vi "SinglePoint-RemoveResultChannel.vi"(8 "Error in":errorcluster, 11 "Custom Device ref":T1 format="%.0x") -> (0 "Error out":errorcluster, 3 "Custom Device ref out":T1 format="%.0x")   [LabVIEW 2017, in "Waveform-Processing-Custom-Device Shared.lvlib" / "SinglePoint.lvlib"]
doc: "This application uses the Result Section group to find and remove output channel of the \"SP\" (Single Point) channel type"
uses:
  SinglePoint.lvlib
  <vilib>/NI Veristand/Custom Device API/Custom Device Item Ref.ctl
  Constants.vi
  <vilib>/NI Veristand/Custom Device API/Get Item Property (Dependent Node Pointer).vi
  System Explorer/Waveform-Processing-Custom-Device System Explorer.lvlib
  <vilib>/NI VeriStand/Custom Device API/Custom Device API.lvlib
  Waveform-Processing-Custom-Device Shared.lvlib
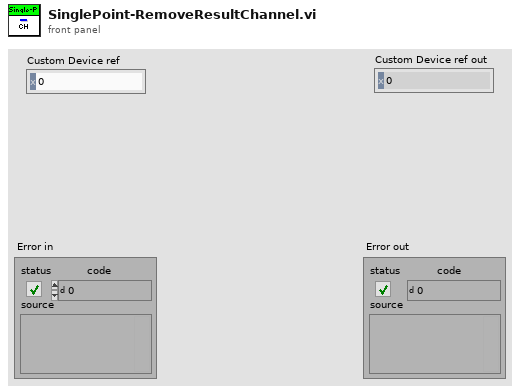
[diagram p1: front panel]
types:
  T1 = typedef "Custom Device API.lvlib/Custom Device Item Ref.ctl" = u64
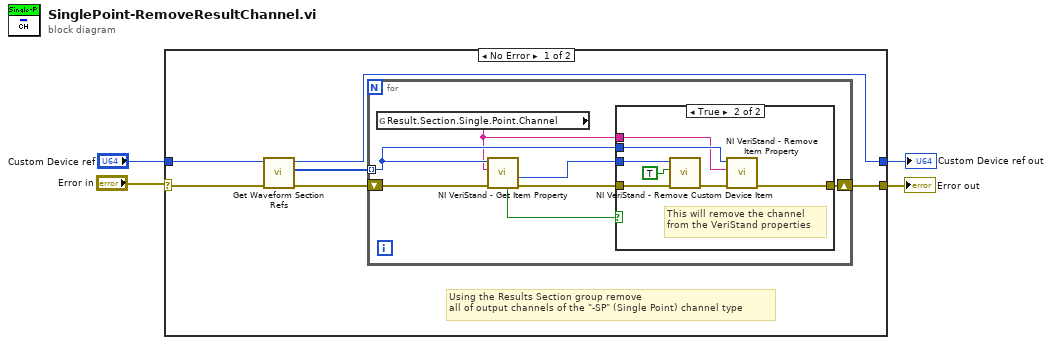
[diagram p0: block diagram]
diagram:
  n1 = case shown="No Error" "Error in" {
    selector: "Error in" -> [w10 w27]
    tunnel: "Custom Device ref" -> [w9 w26]
    tunnel: [w6 w27] -> w3
    tunnel: [w5 w26] -> w1
    frame No Error {
      # "Using the Results Section group remove \nall of output channels of the \"-SP\" (Single Point) channel type"
      n2 = call "Get Waveform Section Refs.vi"("Error in"=w10, "Device Ref in"=w9) -> ("Error out"=w8:errorcluster, "Result Section Refs"=w7:T1[], "Device Ref out"=w5:T1)  [unwired: 7 in]
      n3 = for {
        tunnel: w7 -> [w13] mode=indexing
        shift-right: [w14] -> w6
        shift-left: w8 -> [w17]
        n4 = global read "Constants.vi" "Result.Section.Single.Point.Channel"() -> (w12:string)
        n5 = call-poly <vilib>:"NI VeriStand - Get Item Property.vi"("error in (no error)"=w17, "Property Name"=w12, "Item Ref in"=w13) -> ("error out"=w16:errorcluster, "Dependent Node Ref"=w15:T1, "Found"=w11:bool)  [unwired: 5 in, 1 out]
        n6 = case shown="True" w11 {
          tunnel: w16 -> [w18 w25]
          tunnel: w15 -> [_ w24]
          tunnel: [w18 w21] -> w14
          tunnel: w13 -> [_ w20]
          tunnel: w12 -> [_ w19]
          frame False {
          }
          frame True {
            # "This will remove the channel \nfrom the VeriStand properties"
            n7 = call <vilib>:"NI VeriStand - Remove Custom Device Item.vi"("error in (no error)"=w25, "Force Delete (F)"=TRUE, "Item Ref in"=w24) -> ("error out"=w22:errorcluster)  [unwired: 7 in, 1 out]
            n8 = call <vilib>:"NI VeriStand - Remove Item Property.vi"("error in (no error)"=w22, "Property Name"=w19, "Item Ref in"=w20) -> ("error out"=w21:errorcluster)  [unwired: 6 in, 2 out]
          }
        }
      }
    }
    frame Error {
    }
  }
  "Error out" <- w3
  "Custom Device ref out" <- w1
